vi "LC_WatchDogTimer.vi"() -> ()   [LabVIEW 2016]
uses:
  <vilib>/RTwatchdog.llb/Watchdog status enum.ctl
  <vilib>/RTwatchdog.llb/Watchdog expiration actions.ctl
  LC1_Global.vi
panel:
  in  "expire watchdog":bool
  out "watchdogID out":u64
  out "watchdog status":T1
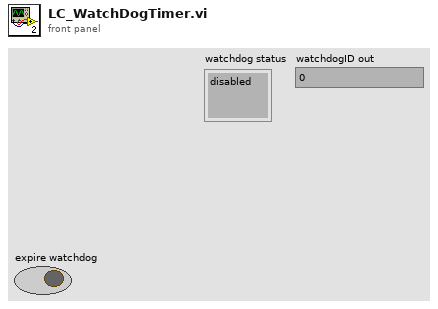
[diagram p1: front panel]
types:
  T1 = typedef "Watchdog status enum.ctl" = enum16{"disabled", "expired", "running"}
  T2 = typedef "Watchdog expiration actions.ctl" = cluster{"reset":bool, "occurrence":bool, "trigger protocol":enum16{"active high", "active low", "open collector"}, "trigger line":enum16{"none", "line 0", "line 1", "line 2", "line 3", "line 4", "line 5", "line 6", "line 7", "SMB line 0"}, "disable watchdog on VI exit":bool}
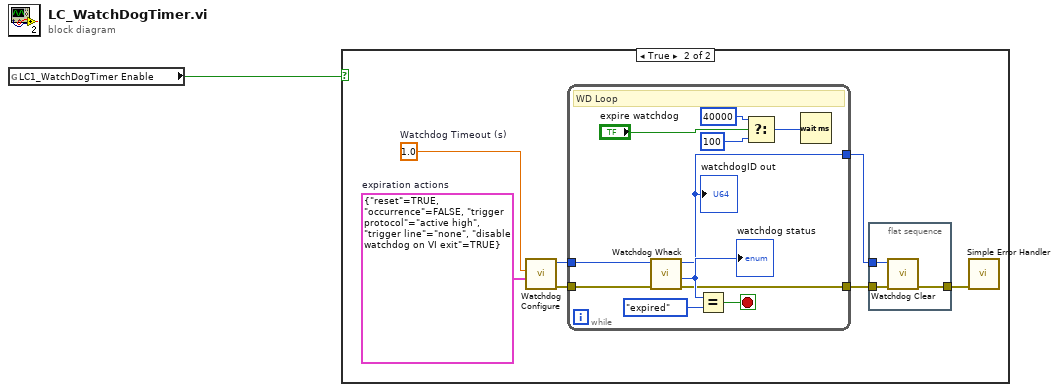
[diagram p0: block diagram]
diagram:
  n1 = global read "LC1_Global.vi" "LC1_WatchDogTimer Enable"() -> (w1:bool)
  n2 = case shown="True" w1 {
    frame False {
    }
    frame True {
      w6 = T2 {"reset"=TRUE, "occurrence"=FALSE, "trigger protocol"=enum."active high", "trigger line"=enum."none", "disable watchdog on VI exit"=TRUE}  # expiration actions
      w8 = 1.0  # Watchdog Timeout (s)
      n3 = call <vilib>:"Watchdog Configure.vi"("expiration actions"=w6, "timeout (1 sec)"=w8) -> ("error out"=w3:errorcluster, "watchdogID"=w7:u64)  [unwired: 2 in, 2 out]
      n4 = while {
        tunnel: w7 -> [w22]
        tunnel: [w18] -> w5
        tunnel: [w17] -> w4
        tunnel: w3 -> [w16]
        stop <- w19 stop-if-true
        # "WD Loop"
        n5 = call <vilib>:"Watchdog Whack.vi"("error in (no error)"=w16, "watchdogID in"=w22) -> ("error out"=w17:errorcluster, "watchdog status"=w20:T1, "watchdogID out"=w18:u64)  [unwired: 3 in]
        "watchdog status" <- w20
        "watchdogID out" <- w18
        n6 = Equal?(x=w20, y=Watchdog_status_enum."expired") -> (x = y?=w19:bool)
        n7 = Select(t=u32 40000 ("wait (msec)"), s="expire watchdog", f=u32 100 ("wait (msec)")) -> (s? t:f=w15:u32)
        n8 = Wait (ms)(milliseconds to wait=w15) -> ()  [unwired: 1 out]
      }
      n9 = flat-sequence {
        tunnel: w4 -> [w11]
        tunnel: w5 -> [w10]
        tunnel: [w9] -> w2
        frame #0 {
          n10 = call <vilib>:"Watchdog Clear.vi"("error in (no error)"=w11, "watchdogID in"=w10) -> ("error out"=w9:errorcluster)  [unwired: 5 in]
        }
      }
      n11 = call <vilib>:"Simple Error Handler.vi"("error in (no error)"=w2) -> ()  [unwired: 4 in, 5 out]
    }
  }
